vi "_USB_CAN_Ver_Trans_.vi"(1 "u16Ver":u16 format="%04x") -> (0 "strVer":string)   [LabVIEW 2011]
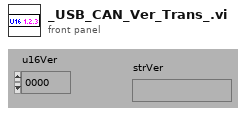
[diagram p1: front panel]
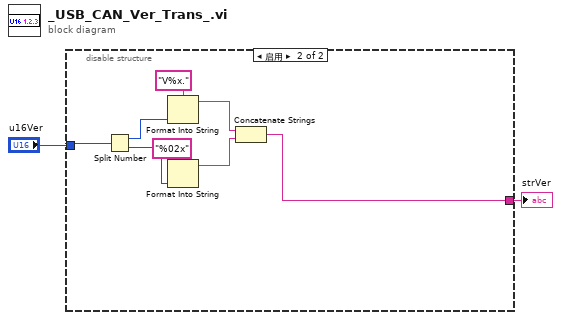
[diagram p0: block diagram]
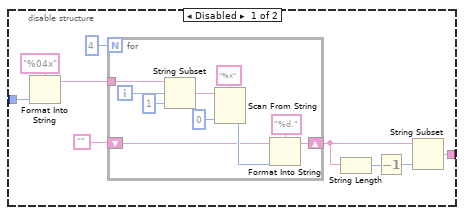
[diagram p2: hidden frame]
diagram:
  n1 = disable-structure shown="启用" {
    disable-tunnel: "u16Ver" -> [w11 w29]
    disable-tunnel: [w3 w22] -> w1
    frame Disabled {
      n2 = Format Into String(format string="%04x" ("格式字符串"), w11) -> (resulting string=w9:string)  [unwired: 2 in, 1 out]
      n3 = for {
        N: 4 -> [_]
        tunnel: w9 -> [w21]
        shift-right: [w12] -> w6
        shift-left: "" -> [w13]
        i -> [w20]
        n4 = String Subset(string=w21, offset (0)=w20, length (rest)=1 ("长度（剩余）")) -> (substring=w18:string)
        n5 = Scan From String(format string="%x" ("格式字符串"), input string=w18, default 1=u8 0 ("默认值 1")) -> (output 1=w15:u8)  [unwired: 2 in, 3 out]
        n6 = Format Into String(format string="%d." ("格式字符串"), initial string=w13, w15) -> (resulting string=w12:string)  [unwired: 1 in, 1 out]
      }
      n7 = String Length(string=w6) -> (length=w5:i32)
      n8 = Decrement(x=w5) -> (x-1=w4:i32)
      n9 = String Subset(string=w6, length (rest)=w4) -> (substring=w3:string)  [unwired: 1 in]
    }
    frame Enabled {
      n10 = Split Number(x=w29) -> (hi(x)=w28:u8, lo(x)=w27:u8)
      n11 = Format Into String(format string="V%x." ("格式字符串"), w28) -> (resulting string=w24:string)  [unwired: 2 in, 1 out]
      n12 = Format Into String(format string="%02x" ("格式字符串"), w27) -> (resulting string=w23:string)  [unwired: 2 in, 1 out]
      n13 = Concatenate Strings(w24, w23) -> (w22:string)
    }
  }
  "strVer" <- w1
